vi "MDAQ_CMD_Write.vi"(5 "milliseconds to wait":u32=50, 7 "CMD":T2=enum."Amplitude", 8 "error in":errorcluster, 9 "Status_Cluster":T1 {"GATESTOP" format="%04x"; "GATESTRT" format="%04x"; "AMPLITUDE" format="%04x"; "M_CYCLES" format="%04x"; "N_CYCLES" format="%04x"; "STEP" format="%04x"; "BASE" format="%04x"; "CHAN" format="%04x"}, 10 "ARG":dbl, 11 "VISA resource name":refnum<visa-resource-name>) -> (0 "error out":errorcluster, 1 "Status_Cluster Out":T1 {"GATESTOP" format="%04x"; "GATESTRT" format="%04x"; "AMPLITUDE" format="%04x"; "M_CYCLES" format="%04x"; "N_CYCLES" format="%04x"; "STEP" format="%04x"; "BASE" format="%04x"; "CHAN" format="%04x"}, 3 "VISA resource name out":refnum<visa-resource-name>)   [LabVIEW 2021]
uses:
  CMD_ARG_Enum.ctl
  Status_Cluster.ctl
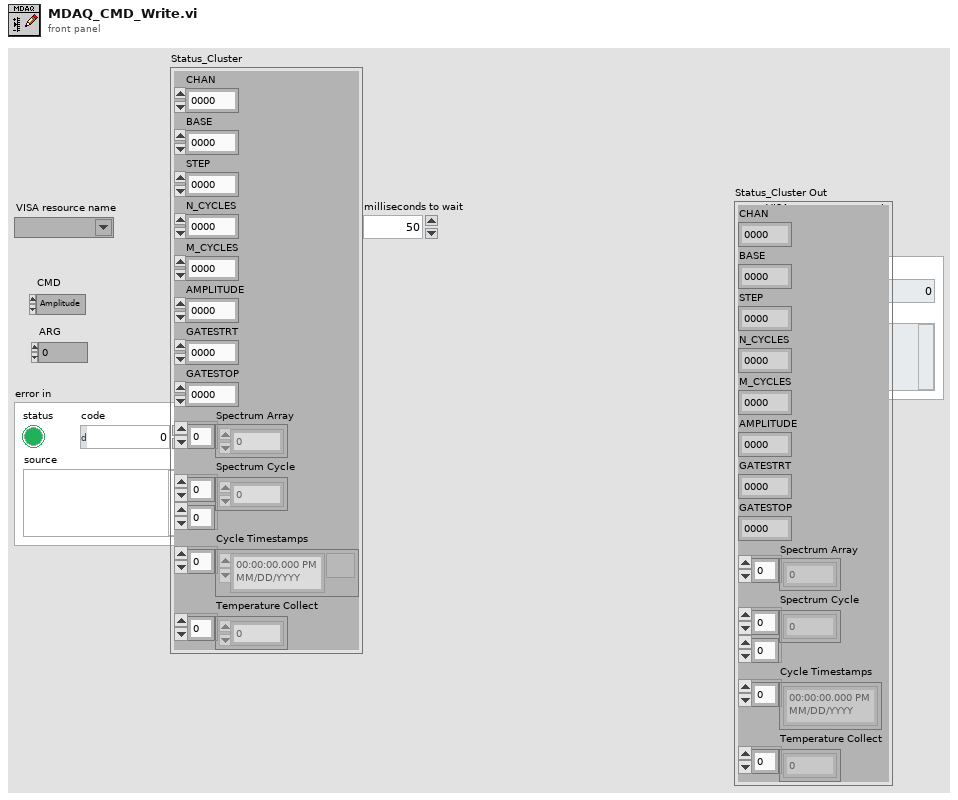
[diagram p1: front panel]
types:
  T1 = typedef "Status_Cluster.ctl" = cluster{"CHAN":u32, "BASE":u32, "STEP":u32, "N_CYCLES":u32, "M_CYCLES":u32, "AMPLITUDE":u32, "GATESTRT":u32, "GATESTOP":u32, "Spectrum Array":u32[], "Spectrum Cycle":u32[][], "Cycle Timestamps":timestamp[], "Temperature Collect":dbl[]}
  T2 = typedef "CMD_ARG_Enum.ctl" = enum16{"N_Cycles", "GateStep", "ASCII_Spectrum", "Waveform", "GateStop", "GateStart", "Amplitude", "Frequency"}
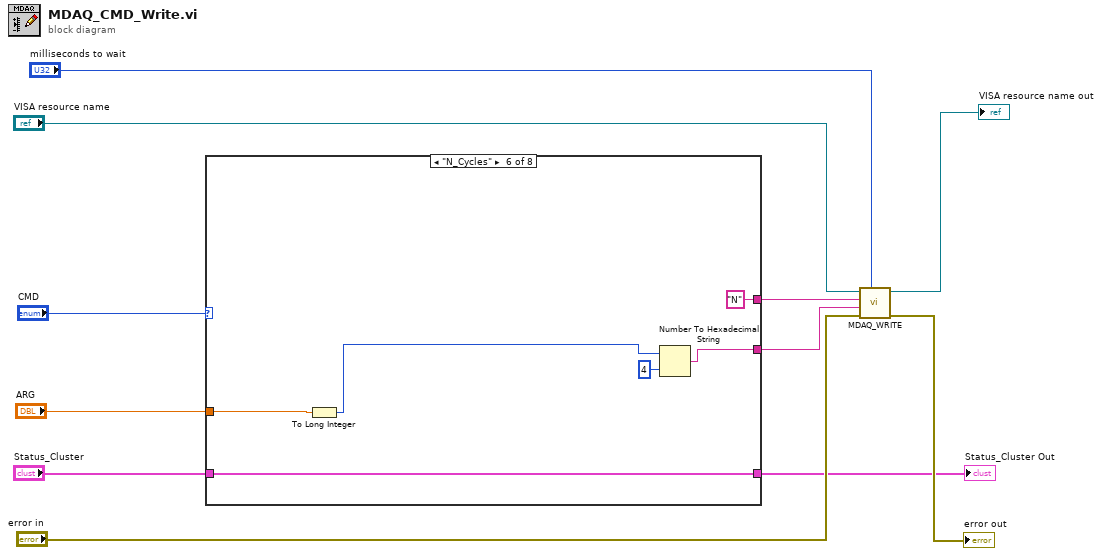
[diagram p0: block diagram]
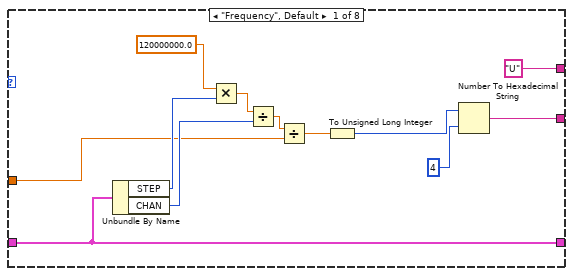
[diagram p2: hidden frame]
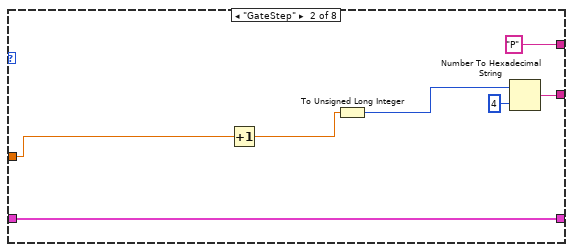
[diagram p3: hidden frame]
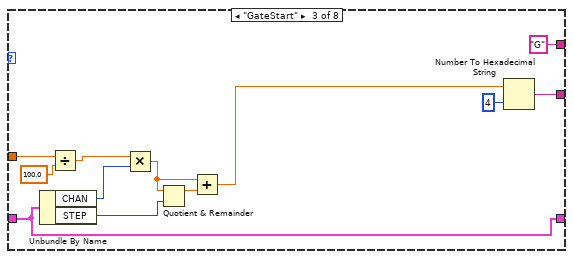
[diagram p4: hidden frame]
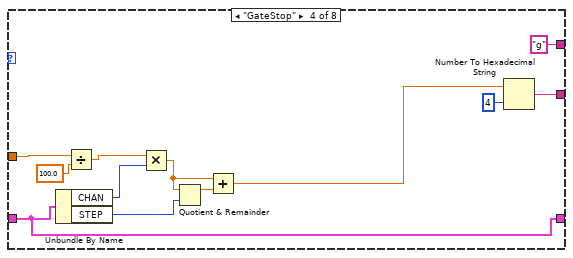
[diagram p5: hidden frame]
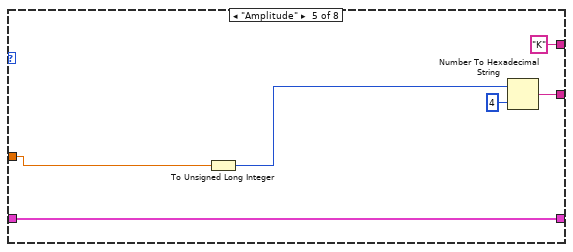
[diagram p6: hidden frame]
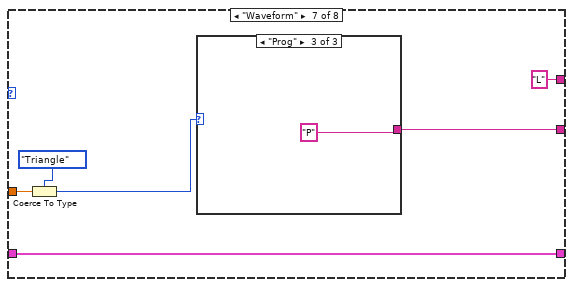
[diagram p7: hidden frame]
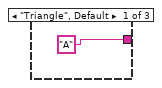
[diagram p8: hidden frame]
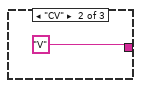
[diagram p9: hidden frame]
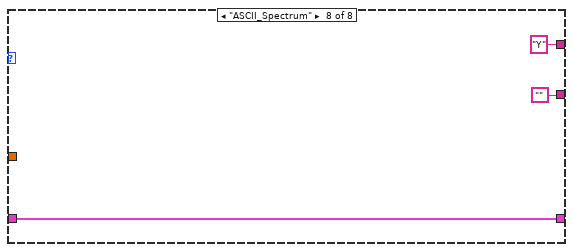
[diagram p10: hidden frame]
diagram:
  n1 = case shown="\"N_Cycles\"" "CMD" {
    tunnel: "ARG" -> [w16 w24 w37 w46 w55 w65 w72 _]
    tunnel: ["U" ("CMD") "P" ("CMD") "G" ("CMD") "g" ("CMD") "K" ("CMD") "N" ("CMD") "L" ("CMD") "Y" ("CMD")] -> w5
    tunnel: [w22 w28 w40 w53 w59 w63 w67 ""] -> w3
    tunnel: "Status_Cluster" -> [w12 w29 w38 w44 w56 w64 w69 w78]
    tunnel: [w12 w29 w38 w44 w56 w64 w69 w78] -> w2
    frame "Frequency", Default {
      n2 = Unbundle By Name(w12) -> ("STEP"=w20:u32, "CHAN"=w18:u32)
      n3 = Multiply(x=120000000.0, y=w20) -> (x*y=w19:dbl)
      n4 = Divide(x=w19, y=w18) -> (x/y=w17:dbl)
      n5 = Divide(x=w17, y=w16) -> (x/y=w15:dbl)
      n6 = To Unsigned Long Integer(number=w15) -> (unsigned 32bit integer=w14:u32)
      n7 = Number To Hexadecimal String(1:i16 4 ("width (-)"), 2:w14) -> (0:w22:string)
    }
    frame "GateStep" {
      n8 = Increment(x=w24) -> (x+1=w25:dbl)
      n9 = To Unsigned Long Integer(number=w25) -> (unsigned 32bit integer=w27:u32)
      n10 = Number To Hexadecimal String(1:i16 4 ("width (-)"), 2:w27) -> (0:w28:string)
    }
    frame "GateStart" {
      n11 = Unbundle By Name(w38) -> ("CHAN"=w41:u32, "STEP"=w35:u32)
      n12 = Divide(x=w37, y=100.0) -> (x/y=w31:dbl)
      n13 = Multiply(x=w31, y=w41) -> (x*y=w33:dbl)
      n14 = Quotient & Remainder(x=w33, y=w35) -> (x-y*floor(x/y)=w34:dbl)  [unwired: 1 out]
      n15 = Add(x=w33, y=w34) -> (x+y=w32:dbl)
      n16 = Number To Hexadecimal String(1:i16 4 ("width (-)"), 2:w32) -> (0:w40:string)
    }
    frame "GateStop" {
      n17 = Unbundle By Name(w44) -> ("CHAN"=w51:u32, "STEP"=w49:u32)
      n18 = Divide(x=w46, y=100.0) -> (x/y=w43:dbl)
      n19 = Multiply(x=w43, y=w51) -> (x*y=w47:dbl)
      n20 = Quotient & Remainder(x=w47, y=w49) -> (x-y*floor(x/y)=w48:dbl)  [unwired: 1 out]
      n21 = Add(x=w47, y=w48) -> (x+y=w45:dbl)
      n22 = Number To Hexadecimal String(1:i16 4 ("width (-)"), 2:w45) -> (0:w53:string)
    }
    frame "Amplitude" {
      n23 = To Unsigned Long Integer(number=w55) -> (unsigned 32bit integer=w58:u32)
      n24 = Number To Hexadecimal String(1:i16 4 ("width (-)"), 2:w58) -> (0:w59:string)
    }
    frame "N_Cycles" {
      n25 = To Long Integer(number=w65) -> (32bit integer=w61:i32)
      n26 = Number To Hexadecimal String(1:i16 4 ("width (-)"), 2:w61) -> (0:w63:string)
    }
    frame "Waveform" {
      n27 = Coerce To Type(0:w72, 1:enum32{"Triangle", "CV", "Prog"}."Triangle" ("Wave Form")) -> (2:w70:enum32{"Triangle", "CV", "Prog"})
      n28 = case shown="\"Prog\"" w70 {
        tunnel: ["A" "V" "P"] -> w67
        frame "Triangle", Default {
        }
        frame "CV" {
        }
        frame "Prog" {
        }
      }
    }
    frame "ASCII_Spectrum" {
    }
  }
  "Status_Cluster Out" <- w2
  n29 = call "MDAQ_WRITE.vi"("milliseconds to wait"="milliseconds to wait", "error in"="error in", "ARG"=w3, "CMD"=w5, "VISA resource name"="VISA resource name") -> ("error out"=→"error out":errorcluster, "VISA resource name out"=→"VISA resource name out":refnum<visa-resource-name>)  [unwired: 5 in]
